vi "ASCII参数转为RTU参数.vi"(1 "ASCII参数":string) -> (0 "RTU参数":string)   [LabVIEW 2015]
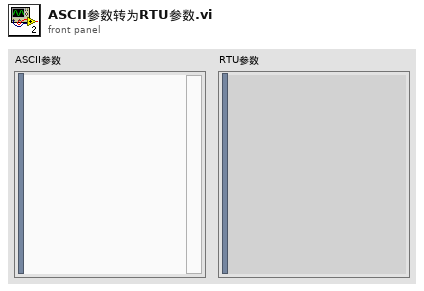
[diagram p1: front panel]
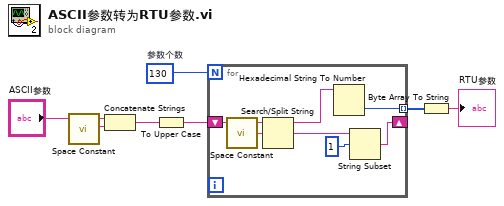
[diagram p0: block diagram]
diagram:
  w5 = 130  # 参数个数
  n1 = call <vilib>:"Space Constant.vi"() -> ("String"=w7:string)
  n2 = Concatenate Strings("ASCII参数", w7) -> (w2:string)
  n3 = To Upper Case(1:w2) -> (0:w1:string)
  n4 = for {
    N: w5 -> [_]
    shift-right: [w11] -> _
    shift-left: w1 -> [w14]
    tunnel: [w8] -> w3 mode=indexing
    n5 = call <vilib>:"Space Constant.vi"() -> ("String"=w13:string)
    n6 = Search/Split String(string=w14, search string/char (-)=w13) -> (substring before match=w9:string, match + rest of string=w12:string)  [unwired: 1 in, 1 out]
    n7 = Hexadecimal String To Number(string=w9) -> (number=w8:u32)  [unwired: 2 in, 1 out]
    n8 = String Subset(string=w12, offset (0)=1 ("偏移量(0)")) -> (substring=w11:string)  [unwired: 1 in]
  }
  n9 = Byte Array To String(unsigned byte array=w3) -> (string=→"RTU参数":string)
